vi "Sleep Until FTE.vi"(8 "error in (no error)":errorcluster, 10 "Wake Time":i64, 11 "CIFCorePlugin in":refnum<class "CIFCorePlugin.lvclass">) -> (0 "error out":errorcluster, 1 "Wake for Houskeeping":bool, 2 "Wake Time (ns)":i64, 3 "CIFCorePlugin out":refnum<class "CIFCorePlugin.lvclass">)   [LabVIEW 2021, in "CIFCorePlugin.lvclass"]
uses:
  CIFCorePlugin.lvclass
  CIFCorePlugin.lvclass/CIFCorePlugin.ctl
  Common/Typedef/Errors.ctl
  <vilib>/CIF Foundation/CIF Utilities/Errors/Append Error Location.vi
  <vilib>/CIF Foundation/CIF Utilities/Time/System Time/LabVIEW Time to TAI Time.vi
  Common/CIFCoreCommon.lvlib
  <vilib>/CIF Foundation/CIF Utilities/Time/Time_CIF_U.lvlib
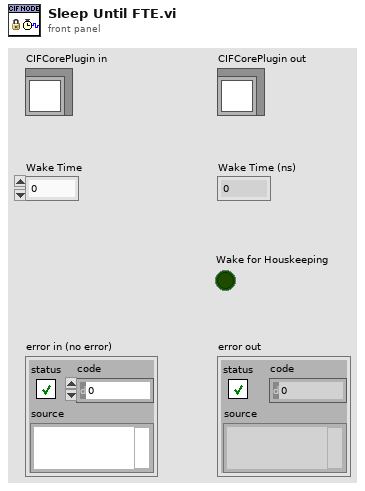
[diagram p1: front panel]
types:
  T1 = typedef "CIFCoreCommon.lvlib/Errors.ctl" = enum16{"Invalid Clock ID", "Long Sleep", "gRPC Server Not Found", "Config Parse", "Timestamp Wrap", "Delayed Execution", "Duplicate Channel", "Missing Channel", "Incorrect Type", "Flatten Error", "Unflatten Data", "Unique Name", "Plugin Not Found", "Plugin Type Not Found", "Plugin Version Not Found", "Manager Not Found", "Numerical Issue", "Time Jump", "Clock ID Match", "Channel Length", "Plugin Connection", "gRPC Server Connection", "PPL Name Match", "Build", "Config Log Parse"}
  T2 = typedef "Time_CIF_U.lvlib/Future Time Event Limits.ctl" = cluster{"Maximum":i64, "Minimum":i64}
  T3 = typedef "Time_CIF_U.lvlib/Clock Conversion Map.ctl" = map{u8, cluster{"Last Reset":i64, "Offset Pair":T4, "Slope":dbl, "1/Slope":dbl}}
  T4 = typedef "Time_CIF_U.lvlib/Timestamp Pair.ctl" = cluster{"System Time":i64, "External Time":i64}
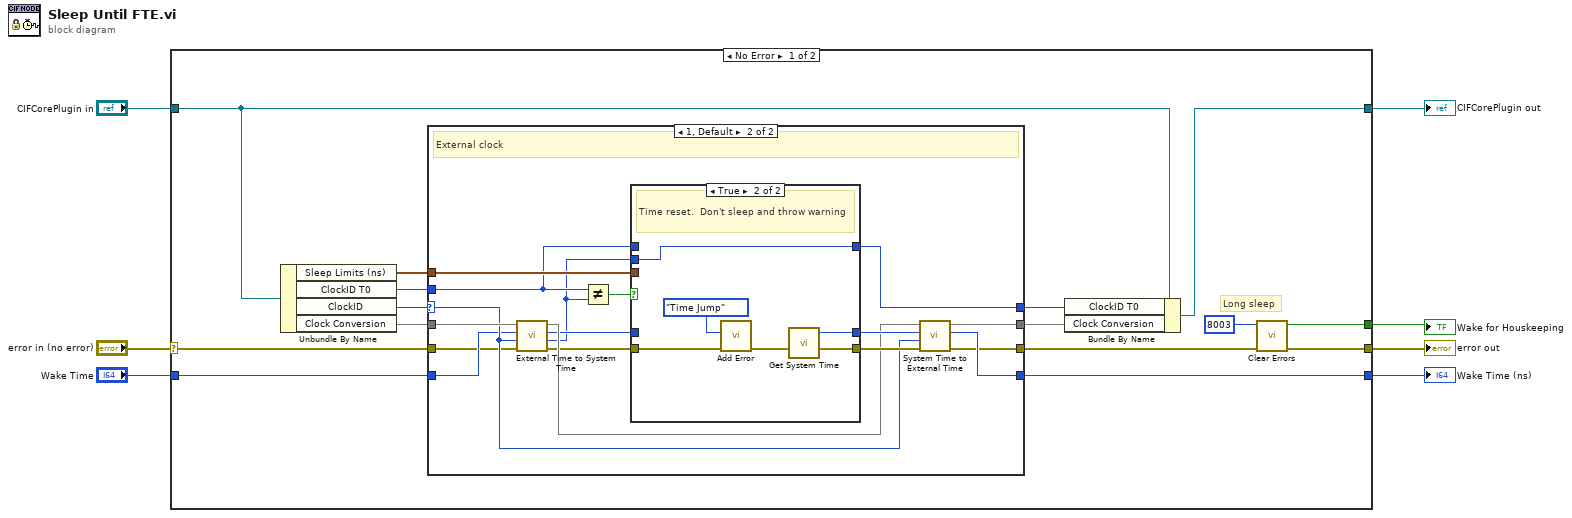
[diagram p0: block diagram]
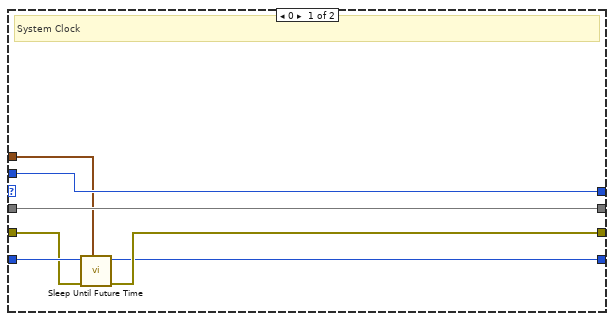
[diagram p2: hidden frame]
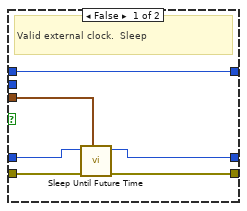
[diagram p3: hidden frame]
diagram:
  n1 = case shown="No Error" "error in (no error)" {
    selector: "error in (no error)" -> [w20 w59]
    tunnel: [w9 w59] -> w6
    tunnel: [w12 w58] -> w4
    tunnel: "CIFCorePlugin in" -> [w16 w58]
    tunnel: "Wake Time" -> [w22 _]
    tunnel: [w11 _] -> w2
    tunnel: [w10 _] -> w1
    frame No Error {
      # "Long sleep"
      n2 = Unbundle By Name(w16) -> ("Sleep Limits (ns)"=w17:T2, "ClockID T0"=w19:i64, "ClockID"=w8:u8, "Clock Conversion"=w21:T3)
      n3 = case shown="1, Default" w8 {
        selector: w8 -> [_ w39]
        tunnel: w22 -> [w27 w38]
        tunnel: w19 -> [w29 w44]
        tunnel: w21 -> [w28 w40]
        tunnel: w20 -> [w26 w34]
        tunnel: [w23 w32] -> w11
        tunnel: [w25 w30] -> w13
        tunnel: w17 -> [w24 w45]
        tunnel: [w28 w31] -> w15
        tunnel: [w29 w43] -> w14
        frame 0 {
          # "System Clock"
          n4 = call <vilib>:"Sleep Until Future Time.vi"("FTE Limits (ns)"=w24, "error in (no error)"=w26, "Wake Time (ns)"=w27) -> ("error out"=w25:errorcluster, "Wake Time (ns)"=w23:i64)  [unwired: 7 in]
        }
        frame 1, Default {
          # "External clock"
          n5 = call <vilib>:"External Time to System Time.vi"("error in (no error)"=w34, "ClockID"=w39, "External Time"=w38, "Clock Convert Map in"=w40) -> ("error out"=w33:errorcluster, "Last Reset Time"=w35:i64, "System Time"=w36:i64, "Clock Convert Map out"=w37:T3)  [unwired: 4 in]
          n6 = Not Equal?(x=w44, y=w35) -> (x != y?=w46:bool)
          n7 = case shown="True" w46 {
            tunnel: w33 -> [w49 w55]
            tunnel: w36 -> [w50 _]
            tunnel: w45 -> [w51 _]
            tunnel: [w48 w54] -> w41
            tunnel: [w47 w53] -> w42
            tunnel: w44 -> [w52 _]
            tunnel: w35 -> [_ w57]
            tunnel: [w52 w57] -> w43
            frame False {
              # "Valid external clock.  Sleep"
              n8 = call <vilib>:"Sleep Until Future Time.vi"("FTE Limits (ns)"=w51, "error in (no error)"=w49, "Wake Time (ns)"=w50) -> ("error out"=w48:errorcluster, "Wake Time (ns)"=w47:i64)  [unwired: 7 in]
            }
            frame True {
              # "Time reset.  Don't sleep and throw warning"
              n9 = call <vilib>:"Add Error.vi"("error in (no error)"=w55, "Error"=Errors."Time Jump") -> ("error out"=w54:errorcluster)  [unwired: 9 in]
              n10 = call <vilib>:"Get System Time.vi"() -> ("Time (ns)"=w53:i64)  [unwired: 5 in]
            }
          }
          n11 = call <vilib>:"System Time to External Time.vi"("error in (no error)"=w41, "ClockID"=w39, "System Time"=w42, "Clock Convert Map in"=w37) -> ("error out"=w30:errorcluster, "External Time"=w32:i64, "Clock Convert Map out"=w31:T3)  [unwired: 4 in, 1 out]
        }
      }
      n12 = Bundle By Name(cluster=w16, "ClockID T0"=w14, "Clock Conversion"=w15) -> (w12:refnum<class "CIFCorePlugin.lvclass">)
      n13 = call <vilib>:"Clear Errors.vi"("error in (no error)"=w13, "specific error code to clear (0: all)"=8003 ("code")) -> ("error out"=w9:errorcluster, "specific error cleared?"=w10:bool)  [unwired: 4 in]
    }
    frame Error {
    }
  }
  "error out" <- w6
  "CIFCorePlugin out" <- w4
  "Wake Time (ns)" <- w2
  "Wake for Houskeeping" <- w1
